vi "4461 - Create IO Channels Parallel Uneven SETTER.vi"(0 "Instrument.Lockin in":refnum<class "Instrument.Lockin.lvclass">, 1 "output terminal configuration":i32, 2 "sample mode":i32, 3 "AO Configuration":T5, 4 "AO":T8 {"AO f (Hz)" min=0.001 max=10000.0; "AO DC (V)" format="%.3p"; "AO Amp (V)" format="%.3p"}, 6 "input terminal configuration":i32, 7 "Channels: Lockin":T15 {"REF phi (°)" format="%#_3g"}, 8 "AI Configuration":T1 {"AI.Coupling" items=["AC"=10045, "DC"=10050, "GND"=10066]}, 9 "AI Buffer Size (S)":i32, 11 "sampling info":cluster{"Fs":dbl, "#s":dbl}) -> (14 "Instrument.Lockin out":refnum<class "Instrument.Lockin.lvclass">)   [LabVIEW 2016, in "Instrument.Lockin.lvclass"]
uses:
  Instrument.Lockin.lvclass
  Typedefs/REF-cluster.ctl
  Typedefs/REF_f-array.ctl
  Typedefs/REF_phi-array.ctl
  Typedefs/AO-cluster.ctl
  Typedefs/AO_Amp-array.ctl
  Typedefs/AO_DC-array.ctl
  Typedefs/AO_f-array.ctl
  Typedefs/AO_phi-array.ctl
  Typedefs/Function-array.ctl
  Typedefs/Function-enum.ctl
  Typedefs/AO.config(UI)-array.ctl
  Typedefs/AO.config(UI)-cluster.ctl
  Typedefs/446xAO-enum.ctl
  Typedefs/AI.config(UI)-array.ctl
  Typedefs/AI.config(UI)-cluster.ctl
  Typedefs/AI.coupling-enum.ctl
  Typedefs/446xAI-enum.ctl
  Instrument.Lockin.lvclass/Instrument.Lockin.ctl
panel:
  # "1"
  # "2"
  # "3"
  # "4"
  # "5"
  # "6"
  # "7"
  # "8"
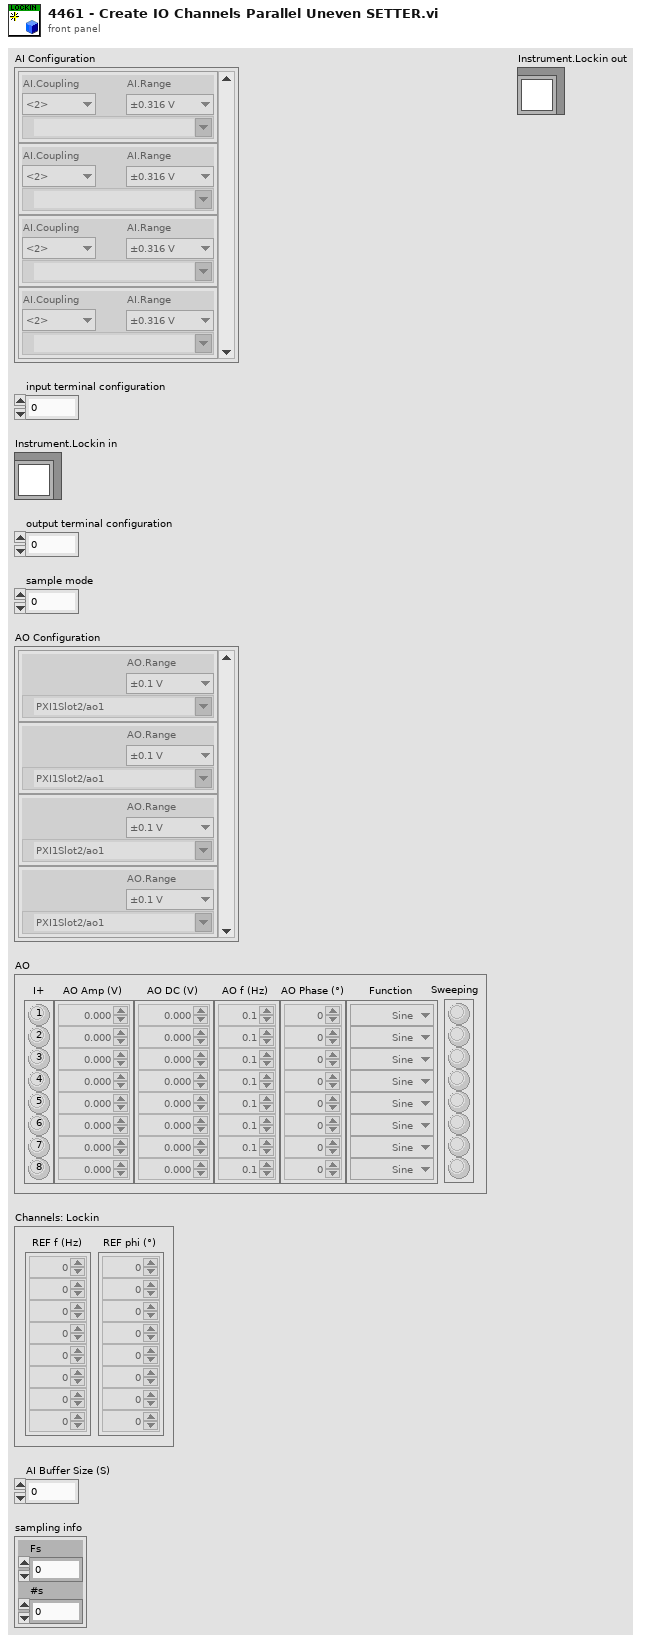
[diagram p1: front panel]
types:
  T1 = typedef "Instrument.Lockin.lvclass/AI.config(UI)-array.ctl" = T2[]
  T2 = typedef "Instrument.Lockin.lvclass/AI.config(UI)-cluster.ctl" = cluster{"AI.Coupling":T3, "AI.channels":tag, "AI.Range":T4}
  T3 = typedef "Instrument.Lockin.lvclass/AI.coupling-enum.ctl" = u16
  T4 = typedef "Instrument.Lockin.lvclass/446xAI-enum.ctl" = enum16{"±0.316 V", "±1.00 V", "±3.16 V", "±10.0 V", "±31.6 V", "±42.4 V"}
  T5 = typedef "Instrument.Lockin.lvclass/AO.config(UI)-array.ctl" = T6[]
  T6 = typedef "Instrument.Lockin.lvclass/AO.config(UI)-cluster.ctl" = cluster{"AO.Range":T7, "AO.channels":tag}
  T7 = typedef "Instrument.Lockin.lvclass/446xAO-enum.ctl" = enum16{"±0.1 V", "±1.0 V", "±10.0 V"}
  T8 = typedef "Instrument.Lockin.lvclass/AO-cluster.ctl" = cluster{"AO Amp (V)":T9, "AO DC (V)":T10, "AO f (Hz)":T11, "AO Phase (°)":T12, "Function":T13, "I+":bool[], "Sweeping":bool[]}
  T9 = typedef "Instrument.Lockin.lvclass/AO_Amp-array.ctl" = dbl[]
  T10 = typedef "Instrument.Lockin.lvclass/AO_DC-array.ctl" = dbl[]
  T11 = typedef "Instrument.Lockin.lvclass/AO_f-array.ctl" = dbl[]
  T12 = typedef "Instrument.Lockin.lvclass/AO_phi-array.ctl" = dbl[]
  T13 = typedef "Instrument.Lockin.lvclass/Function-array.ctl" = T14[]
  T14 = typedef "Instrument.Lockin.lvclass/Function-enum.ctl" = enum16{"Sine", "Triangle", "Square", "Sawtooth"}
  T15 = typedef "Instrument.Lockin.lvclass/REF-cluster.ctl" = cluster{"REF f (Hz)":T16, "REF phi (°)":T17}
  T16 = typedef "Instrument.Lockin.lvclass/REF_f-array.ctl" = dbl[]
  T17 = typedef "Instrument.Lockin.lvclass/REF_phi-array.ctl" = dbl[]
  T18 = typedef "Instrument.Lockin.lvclass/AI.config-array.ctl" = T19[]
  T19 = typedef "Instrument.Lockin.lvclass/AI.config-cluster.ctl" = cluster{"AI.channels":tag, "AI.Coupling":T3, "AI.Range":T4, "input terminal configuration":i32, "DAQ Type":T20}
  T20 = typedef "Instrument.Lockin.lvclass/DAQType-enum.ctl" = enum16{"None", "USB 4431", "PXI 446x"}
  T21 = typedef "Instrument.Lockin.lvclass/AO.config-array.ctl" = T22[]
  T22 = typedef "Instrument.Lockin.lvclass/AO.config-cluster.ctl" = cluster{"AO.channels":tag, "AO.Range":T7, "output terminal configuration":i32, "DAQ Type":T20}
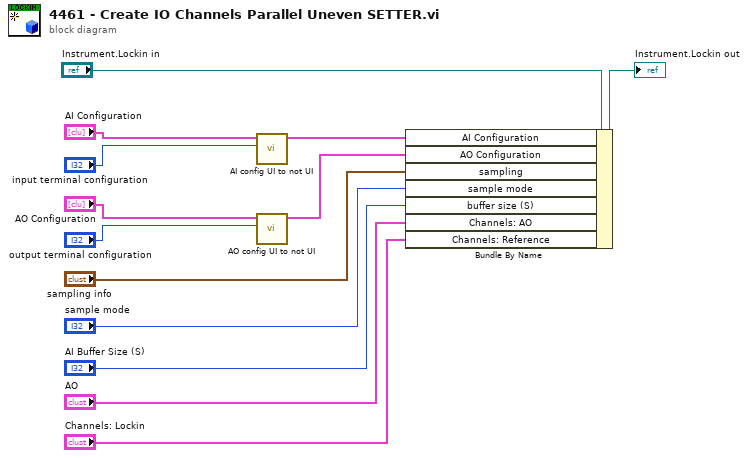
[diagram p0: block diagram]
diagram:
  n1 = call "AI config UI to not UI.vi"("input terminal configuration"="input terminal configuration", "AI Config (UI)"="AI Configuration") -> ("AI Config"=w9:T18)  [unwired: 9 in]
  n2 = call "AO config UI to not UI.vi"("output terminal configuration"="output terminal configuration", "AO Config (UI)"="AO Configuration") -> ("AO Config"=w1:T21)  [unwired: 9 in]
  n3 = Bundle By Name(cluster="Instrument.Lockin in", "AI Configuration"=w9, "AO Configuration"=w1, "sampling"="sampling info", "sample mode"="sample mode", "buffer size (S)"="AI Buffer Size (S)", "Channels: AO"="AO", "Channels: Reference"="Channels: Lockin") -> (→"Instrument.Lockin out":refnum<class "Instrument.Lockin.lvclass">)
